vi "Password Detection New.vi"() -> ()   [LabVIEW 2017]
uses:
  IoT Devices 2/IoT Devices/_subVIs/RWPrefFile.vi
  <vilib>/regexp/Match Regular Expression.xnode
panel:
  in  "Password":string="alohomora"
  out "Door Unlocked":bool
  in  "stop":bool
  out "String":string
  out "error out":errorcluster
  out "Password Approved":bool
  out "Listen For Password":bool caption="boolean"
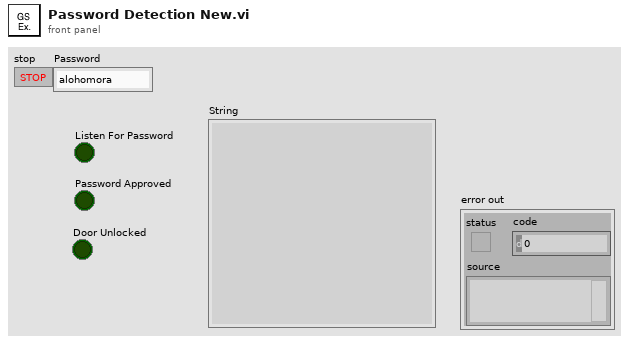
[diagram p1: front panel]
types:
  T1 = typedef "Device.ctl" = cluster{"Device Name":string, "BaseURL":string, "AppKey":string, "Headers":string[], "Timeout":i32, "Identifier":string, "Password":string, "Comments":string, "Handle":u32}
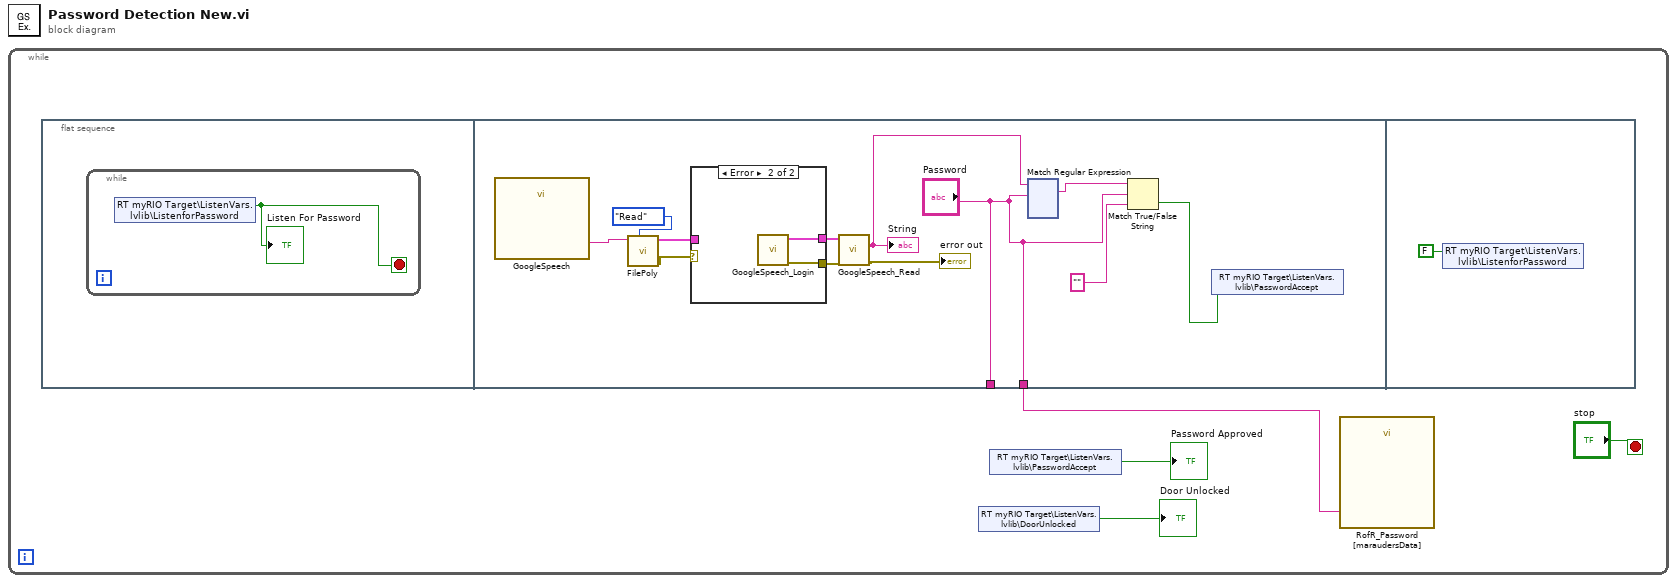
[diagram p0: block diagram]
diagram:
  n1 = while {
    stop <- "stop" stop-if-true
    n2 = flat-sequence {
      tunnel: ["Password"] -> _
      tunnel: ["Password"] -> w1
      frame #0 {
        n3 = while {
          stop <- w5 stop-if-true
          n4 = shared-variable "RT myRIO Target\\ListenVars.lvlib\\ListenforPassword"() -> (w5:bool)  [unwired: 1 in, 1 out]
          "Listen For Password" <- w5
        }
      }
      frame #1 {
        n5 = call "GoogleSpeech"() -> ("Name"=w13:string)  [unwired: 11 in]
        n6 = call-poly "FilePoly.vi"("Task"=enum16{"Read", "Write"}."Read", "Device Name"=w13) -> ("error out"=w15:errorcluster, "Device Out"=w14:T1)  [unwired: 7 in, 1 out]
        n7 = case shown="Error" w15 {
          selector: w15 -> [w132 _]
          tunnel: [w132 w134] -> w11
          tunnel: [w133 w135] -> w12
          tunnel: w14 -> [w133 _]
          frame No Error {
          }
          frame Error {
            n8 = call "GoogleSpeech_Login.vi"() -> ("error out"=w134:errorcluster, "Device Out"=w135:T1)  [unwired: 10 in]
          }
        }
        n9 = call "GoogleSpeech_Read.vi"("error in"=w11, "Device In"=w12) -> ("error out"=→"error out":errorcluster, "String"=w8:string)  [unwired: 7 in, 1 out]
        "String" <- w8
        n10 = xnode "Match Regular Expression"("input string"=w8, "regular expression"="Password") -> ("whole match"=w10:string)  [unwired: 4 in, 4 out]
        n11 = Match True/False String(2:"" ("false string"), 3:"Password", 4:w10) -> (0:w7:bool)  [unwired: 1 out]
        n12 = shared-variable "RT myRIO Target\\ListenVars.lvlib\\PasswordAccept"(w7) -> ()  [unwired: 1 in, 1 out]
      }
      frame #2 {
        n13 = shared-variable "RT myRIO Target\\ListenVars.lvlib\\ListenforPassword"(FALSE ("ListenforPassword")) -> ()  [unwired: 1 in, 1 out]
      }
    }
    n14 = shared-variable "RT myRIO Target\\ListenVars.lvlib\\DoorUnlocked"() -> (→"Door Unlocked":bool)  [unwired: 1 in, 1 out]
    n15 = shared-variable "RT myRIO Target\\ListenVars.lvlib\\PasswordAccept"() -> (→"Password Approved":bool)  [unwired: 1 in, 1 out]
    n16 = call "RofR_Password [maraudersData]"("string"=w1) -> ()  [unwired: 10 in, 1 out]
  }
